vi "SA40144D.20210128 Device vs BG.vi"() -> ()   [LabVIEW 2020]
uses:
  <userlib>/LevyLab/LV to ITX/Data/Data.lvclass
  <vilib>/Analysis/NI_AALPro.lvlib
panel:
  out "T vs t":cluster{dbl[], dbl[]}(graph)
  out "Decay (uS/hr)":dbl
  out "Conductance (uS)":dbl
  out "G4T vs t":cluster{dbl[], dbl[]}[](graph)
  in  "Path":path
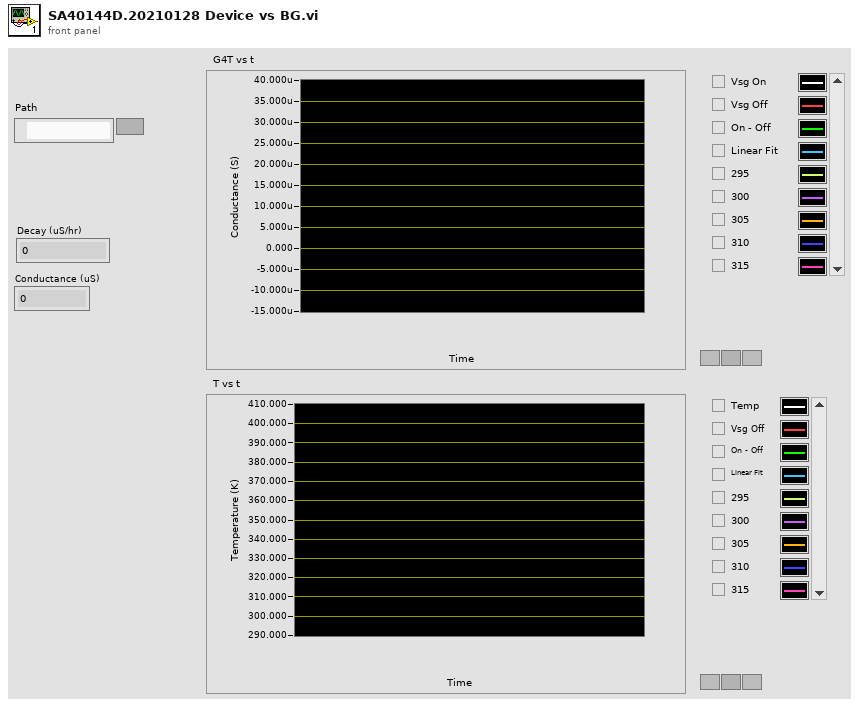
[diagram p1: front panel]
types:
  T1 = typedef "Data.lvclass/Dictionary--cluster.ctl" = cluster{"key":string, "value":variant}
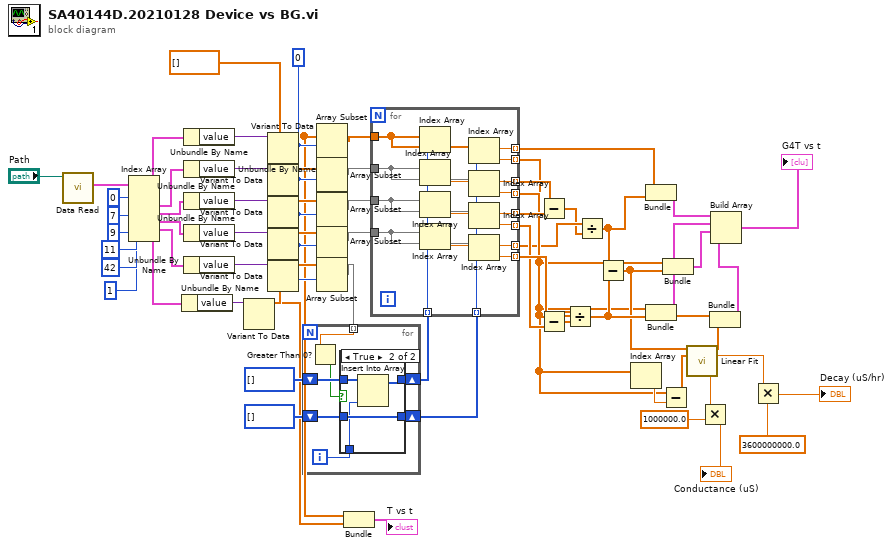
[diagram p0: block diagram]
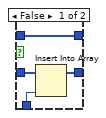
[diagram p2: hidden frame]
diagram:
  w8 = 0
  w4 = dbl[] []
  n1 = call <userlib>:"Data Read.vi"("path"="Path") -> ("Data (Dictionary)"=w64:T1[])  [unwired: 7 in, 3 out]
  n2 = Index Array(array=w64, index #1=0 ("index"), index #2=7 ("index"), index #3=9 ("index"), index #4=11 ("index"), index #5=42 ("index"), index #6=1) -> (element #1=w55:T1, element #2=w58:T1, element #3=w59:T1, element #4=w57:T1, element #5=w56:T1, element #6=w6:T1)
  n3 = Unbundle By Name(w6) -> ("value"=w5:variant)
  n4 = Unbundle By Name(w55) -> ("value"=w54:variant)
  n5 = Unbundle By Name(w58) -> ("value"=w51:variant)
  n6 = Unbundle By Name(w59) -> ("value"=w50:variant)
  n7 = Unbundle By Name(w57) -> ("value"=w52:variant)
  n8 = Unbundle By Name(w56) -> ("value"=w53:variant)
  n9 = Variant To Data(type=w4, Variant=w5) -> (data=w3:dbl[])  [unwired: 1 in, 1 out]
  n10 = Variant To Data(type=w4, Variant=w54) -> (data=w2:dbl[])  [unwired: 1 in, 1 out]
  n11 = Variant To Data(type=w4, Variant=w51) -> (data=w28:dbl[])  [unwired: 1 in, 1 out]
  n12 = Variant To Data(type=w4, Variant=w50) -> (data=w29:dbl[])  [unwired: 1 in, 1 out]
  n13 = Variant To Data(type=w4, Variant=w52) -> (data=w30:dbl[])  [unwired: 1 in, 1 out]
  n14 = Variant To Data(type=w4, Variant=w53) -> (data=w31:dbl[])  [unwired: 1 in, 1 out]
  n15 = Array Subset(array=w2, index=w8) -> (w27:dbl[])  [unwired: 1 in]
  n16 = Array Subset(array=w28, index=w8) -> (w26:dbl[])  [unwired: 1 in]
  n17 = Array Subset(array=w29, index=w8) -> (w25:dbl[])  [unwired: 1 in]
  n18 = Array Subset(array=w30, index=w8) -> (w24:dbl[])  [unwired: 1 in]
  n19 = Array Subset(array=w31, index=w8) -> (w9:dbl[])  [unwired: 1 in]
  n20 = for {
    shift-right: [w71] -> w47
    shift-left: i32[] [] -> [w69]
    shift-right: [w70] -> w46
    shift-left: i32[] [] -> [w68]
    tunnel: w9 -> [w66] mode=indexing
    i -> [w72]
    n21 = Greater Than 0?(x=w66) -> (x > 0?=w67:bool)
    n22 = case shown="True" w67 {
      tunnel: w72 -> [w73 w77]
      tunnel: [w76 w79] -> w71
      tunnel: [w75 w80] -> w70
      tunnel: w69 -> [w76 w78]
      tunnel: w68 -> [w74 w80]
      frame False {
        n23 = Insert Into Array(array=w74, new element=w73) -> (w75:i32[])  [unwired: 1 in]
      }
      frame True {
        n24 = Insert Into Array(array=w78, new element=w77) -> (w79:i32[])  [unwired: 1 in]
      }
    }
  }
  n25 = Bundle(w2, w3) -> (→"T vs t":cluster{dbl[], dbl[]})  [unwired: 1 in]
  n26 = for {
    tunnel: w47 -> [w94] mode=indexing
    tunnel: w46 -> [w93] mode=indexing
    tunnel: w26 -> [w90]
    tunnel: w27 -> [w89]
    tunnel: w25 -> [w91]
    tunnel: w24 -> [w92]
    tunnel: [w88] -> w45 mode=indexing
    tunnel: [w87] -> w39 mode=indexing
    tunnel: [w86] -> w43 mode=indexing
    tunnel: [w85] -> w41 mode=indexing
    tunnel: [w84] -> w42 mode=indexing
    tunnel: [w83] -> w44 mode=indexing
    tunnel: [w82] -> w22 mode=indexing
    tunnel: [w81] -> w17 mode=indexing
    n27 = Index Array(array=w89, index=w94) -> (element=w82:dbl)
    n28 = Index Array(array=w90, index=w94) -> (element=w83:dbl)
    n29 = Index Array(array=w91, index=w94) -> (element=w86:dbl)
    n30 = Index Array(array=w92, index=w94) -> (element=w87:dbl)
    n31 = Index Array(array=w89, index=w93) -> (element=w81:dbl)
    n32 = Index Array(array=w90, index=w93) -> (element=w84:dbl)
    n33 = Index Array(array=w91, index=w93) -> (element=w85:dbl)
    n34 = Index Array(array=w92, index=w93) -> (element=w88:dbl)
  }
  n35 = Subtract(x=w44, y=w43) -> (x-y=w38:dbl[])
  n36 = Subtract(x=w42, y=w41) -> (x-y=w40:dbl[])
  n37 = Divide(x=w45, y=w40) -> (x/y=w33:dbl[])
  n38 = Divide(x=w39, y=w38) -> (x/y=w34:dbl[])
  n39 = Subtract(x=w34, y=w33) -> (x-y=w23:dbl[])
  n40 = Index Array(array=w17) -> (element=w21:dbl)  [unwired: 1 in]
  n41 = Bundle(w22, w34) -> (w36:cluster{dbl[], dbl[]})  [unwired: 1 in]
  n42 = Bundle(w17, w33) -> (w37:cluster{dbl[], dbl[]})  [unwired: 1 in]
  n43 = Subtract(x=w17, y=w21) -> (x-y=w20:dbl[])
  n44 = Bundle(w17, w23) -> (w32:cluster{dbl[], dbl[]})  [unwired: 1 in]
  n45 = call <vilib>:"Linear Fit.vi"("Y"=w23, "X"=w20) -> ("Best Linear Fit"=w16:dbl[], "slope"=w19:dbl, "intercept"=w18:dbl)  [unwired: 9 in, 2 out]
  n46 = Multiply(x=w18, y=1000000.0) -> (x*y=→"Conductance (uS)":dbl)
  n47 = Bundle(w17, "Best Linear Fit"=w16) -> (w15:cluster{dbl[], "Best Linear Fit":dbl[]})  [unwired: 1 in]
  n48 = Build Array(w36, w37, w32, w15) -> (→"G4T vs t":cluster{dbl[], "Best Linear Fit":dbl[]}[])
  n49 = Multiply(x=w19, y=3600000000.0) -> (x*y=→"Decay (uS/hr)":dbl)
